vi "Table Clear.vi"(8 "Error (In)":errorcluster, 9 "Lvdt":refnum<vi>, 10 "Load":refnum<vi>, 11 "Table (In)":refnum<vi>) -> (0 "Error (Out)":errorcluster, 3 "Table (Out)":refnum<vi>)   [LabVIEW 2015]
panel:
  out "error out 2":errorcluster
  out "error out":errorcluster
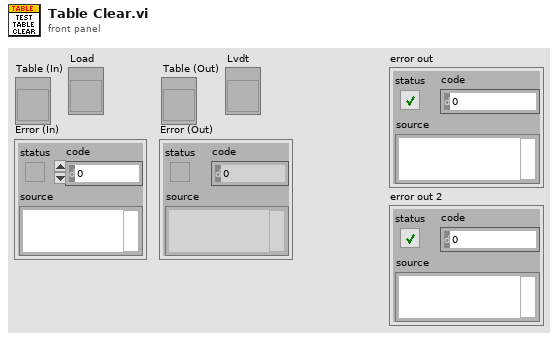
[diagram p1: front panel]
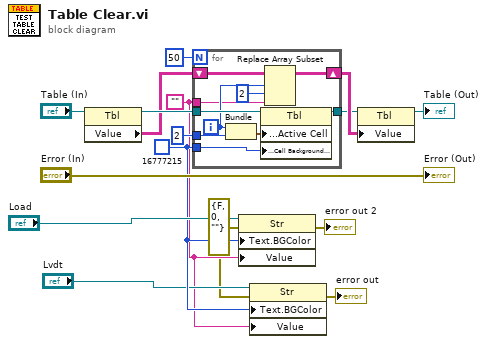
[diagram p0: block diagram]
diagram:
  w1 = errorcluster {"status"=FALSE, "code"=0, "source"=""} ("error in (no error)")
  w4 = ""
  w6 = u32 16777215
  n1 = property class="Tbl"(reference="Table (In)") -> (reference out=w13:refnum<vi>, "Value"=w11:string[][])  [unwired: 1 in, 1 out]
  n2 = for {
    N: 50 -> [_]
    tunnel: w6 -> [w25]
    tunnel: 2 -> [w24]
    tunnel: w13 -> [w23]
    tunnel: [w22] -> w8
    tunnel: w4 -> [w19]
    shift-right: [w17] -> w10
    shift-left: w11 -> [w18]
    i -> [w21]
    n3 = Bundle(w21, w24) -> (w26:cluster{i32, i32})  [unwired: 1 in]
    n4 = property class="Tbl"(reference=w23, "Active Cell:Active Cell"=w26, "Active Cell:Cell Background Color"=w25) -> (reference out=w22:refnum<vi>)  [unwired: 1 in, 1 out]
    n5 = Replace Array Subset(array=w18, new element=w19, index (row)=w21, index (col)=2 ("disabled index (col)")) -> (w17:string[][])
  }
  n6 = property class="Str"(reference="Load", error in=w1, "Text.BGColor"=w6, "Value"=w4) -> (error out=→"error out 2":errorcluster)  [unwired: 1 out]
  n7 = property class="Str"(reference="Lvdt", error in=w1, "Text.BGColor"=w6, "Value"=w4) -> (error out=→"error out":errorcluster)  [unwired: 1 out]
  n8 = property class="Tbl"(reference=w8, "Value"=w10) -> (reference out=→"Table (Out)":refnum<vi>)  [unwired: 1 in, 1 out]
  "Error (Out)" <- "Error (In)"
